vi "test-trapezoid-profile-execute.vi"() -> (3 "Test Passed":bool)   [LabVIEW 2019]
uses:
  <vilib>/Rock Robotics/WPI/ThirdParty/JAS_Junk/TrajLib/Trajectory_Library.lvlib
  <vilib>/Rock Robotics/WPI/ThirdParty/JAS_Junk/TrajLib/LinearFilter_LP_BW1_Execute.vi
panel:
  out "ApproxEquals 2":bool
  out "ApproxEquals":bool
  out "LibUsage_ProfiledPID":i32 format="%20.0f"
  out "LibUsage_PIDController":i32 format="%20.0f"
  out "LibUsage_Odometry":i32 format="%20.0f"
  out "LibUsage_LinearFIlter":i32 format="%20.0f"
  out "LibUsage_TrapezoidProfile":i32 format="%20.0f"
  out "LibUsage_Kinematics":i32 format="%20.0f"
  out "ActVel":dbl
  out "ActAccel":dbl
  out "ElapsedTIme":dbl format="%20.6f"
  in  "Position\nGoal":dbl=2.0 format="%#_13g"
  out "EstTimeLeft":dbl format="%23.3f"
  out "VelocityDmd":dbl
  out "PositionDmd":dbl
  out "Waveform Chart":T1(graph)
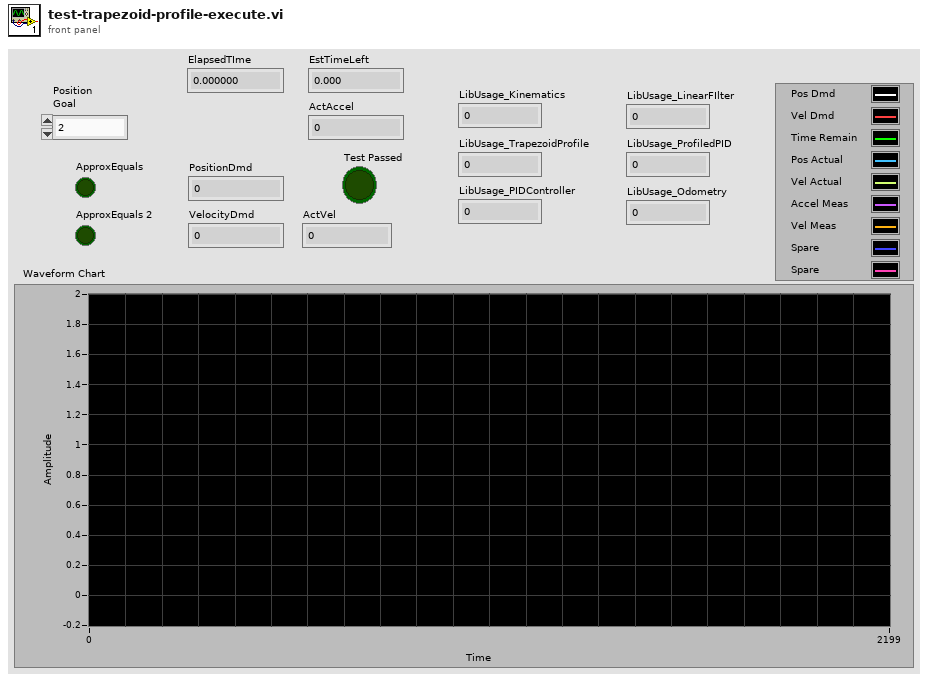
[diagram p1: front panel]
types:
  T1 = cluster{"PositionDmd":dbl, "VelocityDmd":dbl, "EstTimeLeft":dbl, "Output":dbl, "Output":dbl, dbl, dbl, dbl, dbl}
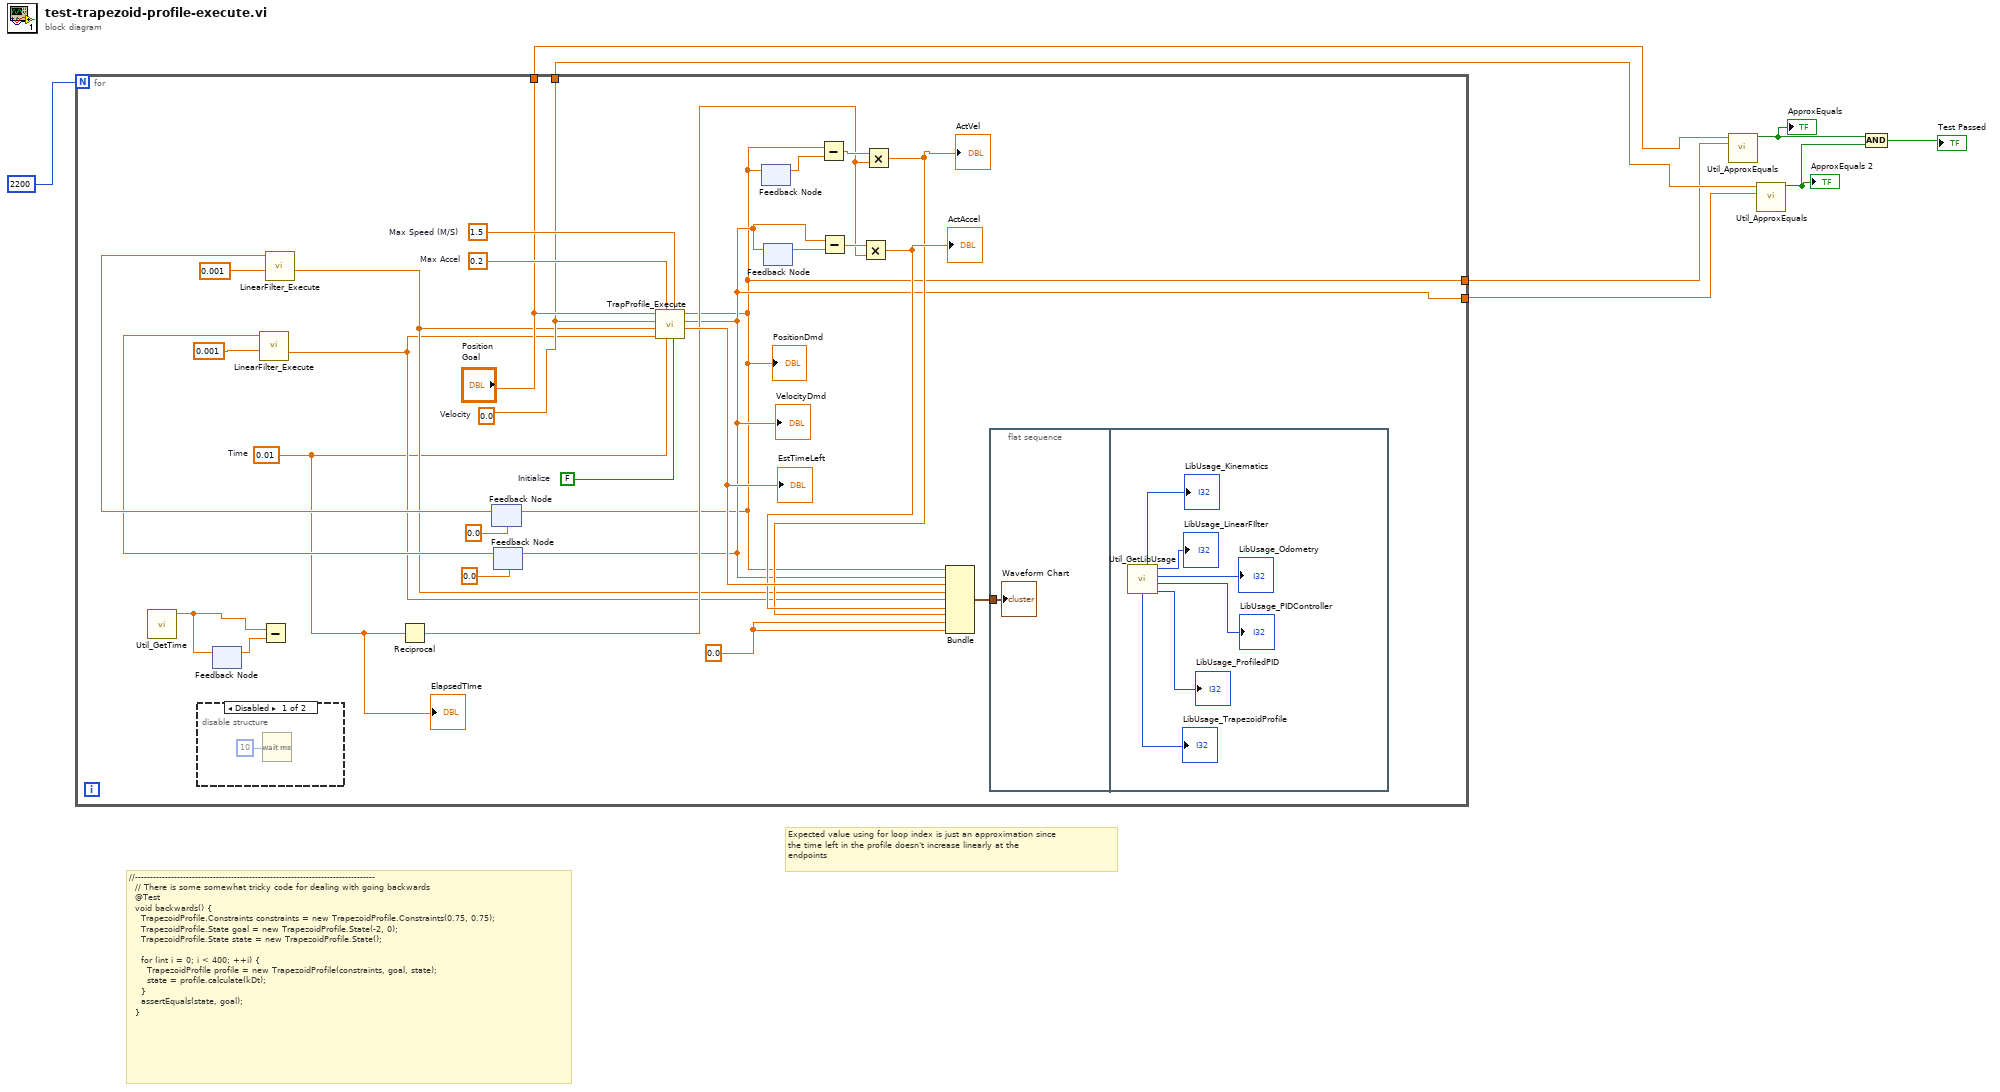
[diagram p0: block diagram]
diagram:
  # "Expected value using for loop index is just an approximation since\nthe time left in the profile doesn't increase linearly at the\nendpoints"
  # "//--------------------------------------------------------------------------------\n  // There is some somewhat tricky code for dealing with going backwards\n  @Test\n  void backwards() {\n    TrapezoidProfile.Constraints constraints = new TrapezoidProfile.Constraints(0.75, 0.75);\n    TrapezoidProfile.State goal = new TrapezoidProfile.State(-2, 0);\n    TrapezoidProfile.State state = new TrapezoidProfile.State();\n\n    for (int i = 0; i < 400; ++i) {\n      TrapezoidProfile profile = new TrapezoidProfile(constraints, goal, state);\n      state = profile.calculate(kDt);\n    }\n    assertEquals(state, goal);\n  }"
  n1 = for {
    N: 2200 -> [_]
    tunnel: ["Position\nGoal"] -> w4
    tunnel: [w15] -> w3
    tunnel: [w12] -> w2
    tunnel: [w18] -> w1
    w17 = FALSE  # Initialize
    w25 = 0.0
    w15 = 0.0  # Velocity
    w35 = 0.2  # Max Accel
    w36 = 1.5  # Max Speed (M/S)
    w11 = 0.01  # Time
    n2 = call <vilib>:"Util_GetTime.vi"() -> ("FPGA_Time_Seconds"=w28:dbl)  [unwired: 9 in, 2 out]
    n3 = disable-structure shown="Disabled" {
      frame Disabled {
        n4 = Wait (ms)(milliseconds to wait=u32 10) -> ()  [unwired: 1 out]
      }
      frame Enabled {
      }
    }
    n5 = feedback-in #1(w28) -> ()
    n6 = feedback #1() -> (w27:dbl)  [unwired: 1 in]
    n7 = Subtract(x=w28, y=w27) -> ()  [unwired: 1 out]
    n8 = Reciprocal(x=w11) -> (1/x=w19:dbl)
    n9 = feedback #2(0.0 ("PositionDmd")) -> (w34:dbl)
    n10 = call-poly <vilib>:"LinearFilter_Execute.vi"("TimeConstant"=0.001, "Input"=w34) -> ("Output"=w14:dbl)  [unwired: 9 in]
    n11 = feedback #3(0.0 ("VelocityDmd")) -> (w33:dbl)
    n12 = call-poly <vilib>:"LinearFilter_Execute.vi"("TimeConstant"=0.001, "Input"=w33) -> ("Output"=w13:dbl)  [unwired: 9 in]
    n13 = call <vilib>:"TrapProfile_Execute.vi"("Initialize"=w17, "Max Speed"=w36, "TimePeriod"=w11, "Max Accel"=w35, "CurrentVelocity"=w13, "CurrentPosition"=w14, "GoalVelocity"=w15, "GoalPosition"="Position\nGoal") -> ("EstTimeLeft"=w32:dbl, "VelocityDmd"=w18:dbl, "PositionDmd"=w12:dbl)  [unwired: 1 out]
    "PositionDmd" <- w12
    "VelocityDmd" <- w18
    "EstTimeLeft" <- w32
    n14 = feedback-in #2(w12) -> ()
    n15 = feedback-in #3(w18) -> ()
    n16 = feedback #4() -> (w24:dbl)  [unwired: 1 in]
    n17 = feedback-in #4(w12) -> ()
    n18 = feedback #5() -> (w26:dbl)  [unwired: 1 in]
    n19 = feedback-in #5(w18) -> ()
    n20 = Subtract(x=w12, y=w24) -> (x-y=w21:dbl)
    n21 = Subtract(x=w18, y=w26) -> (x-y=w20:dbl)
    n22 = Multiply(x=w20, y=w19) -> (x*y=w23:dbl)
    "ActAccel" <- w23
    n23 = Multiply(x=w21, y=w19) -> (x*y=w22:dbl)
    "ActVel" <- w22
    n24 = Bundle("PositionDmd"=w12, "VelocityDmd"=w18, "EstTimeLeft"=w32, "Output"=w14, "Output"=w13, w23, w22, w25, w25) -> (w31:T1)  [unwired: 1 in]
    n25 = flat-sequence {
      tunnel: w31 -> [w38]
      frame #0 {
        "Waveform Chart" <- w38
      }
      frame #1 {
        n26 = call <vilib>:"Util_GetLibUsage.vi"() -> ("LibUsage_ProfiledPID"=→"LibUsage_ProfiledPID":i32, "LibUsage_PIDController"=→"LibUsage_PIDController":i32, "LibUsage_Odometry"=→"LibUsage_Odometry":i32, "LibUsage_LinearFIlter"=→"LibUsage_LinearFIlter":i32, "LibUsage_TrapezoidProfile"=→"LibUsage_TrapezoidProfile":i32, "LibUsage_Kinematics"=→"LibUsage_Kinematics":i32)  [unwired: 6 in]
      }
    }
    "ElapsedTIme" <- w11
  }
  n27 = call <vilib>:"Util_ApproxEquals.vi"("Value 2"=w2, "Value 1"=w4) -> ("ApproxEquals"=w6:bool)  [unwired: 9 in]
  "ApproxEquals" <- w6
  n28 = call <vilib>:"Util_ApproxEquals.vi"("Value 2"=w1, "Value 1"=w3) -> ("ApproxEquals"=w5:bool)  [unwired: 9 in]
  "ApproxEquals 2" <- w5
  n29 = And(x=w6, y=w5) -> (x .and. y?=→"Test Passed":bool)
